vi "SetRef.vi"(8 "error in (no error)":errorcluster, 10 "Set External":bool, 11 "SpecA_ESA in":refnum<class "SpecA_ESA.lvclass">) -> (0 "error out":errorcluster, 3 "SpecA_ESA out":refnum<class "SpecA_ESA.lvclass">)   [LabVIEW 2014, in "SpecA_ESA.lvclass"]
uses:
  SpecA_ESA.lvclass
  SpecA_ESA.lvclass/SpecA_ESA.ctl
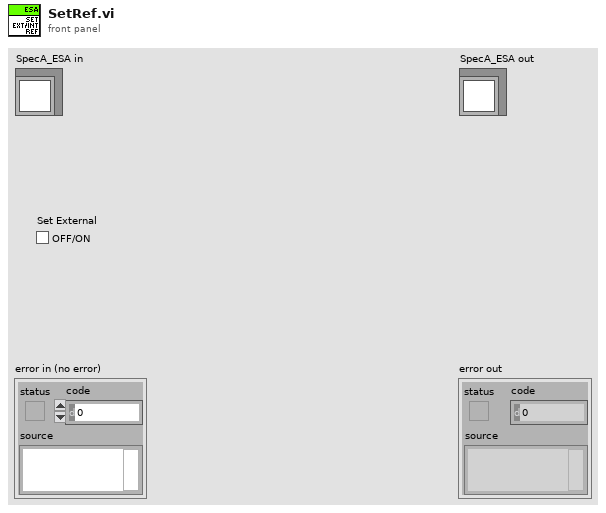
[diagram p1: front panel]
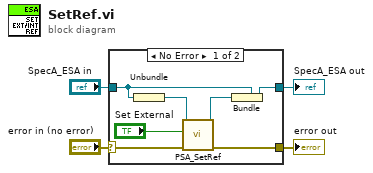
[diagram p0: block diagram]
diagram:
  n1 = case shown="No Error" "error in (no error)" {
    selector: "error in (no error)" -> [w5 w13]
    tunnel: [w9 w12] -> w4
    tunnel: "SpecA_ESA in" -> [w8 w12]
    tunnel: [w6 w13] -> w2
    frame No Error {
      n2 = Unbundle(w8) -> (w10:refnum<visa-resource-name>)
      n3 = call "PSA_SetRef.vi"("error in (no error)"=w5, "Set External"="Set External", "VISA resource name"=w10) -> ("error out"=w6:errorcluster, "VISA resource name out"=w7:refnum<visa-resource-name>)  [unwired: 7 in]
      n4 = Bundle(cluster=w8, w7) -> (w9:refnum<class "SpecA_ESA.lvclass">)
    }
    frame Error {
    }
  }
  "error out" <- w2
  "SpecA_ESA out" <- w4
